vi "PantherLAB_Log - Rename DQMH Event.vi"(9 "New Event Name":string, 10 "Event Info (Existing)":T1={"Event VI Path"=path "", "Argument Path"=path "", "Wait Argument Path"=path "", "Event Arg Owner"=-1, "Event Name"="", "Type"=enum."Request"}, 11 "Module Info":T3) -> (0 "error out":errorcluster)   [LabVIEW 2016]
doc: "_____\nCreated using DQMH Framework: Event Scripter 7.1.0.1450."
uses:
  <vilib>/Delacor/Delacor QMH/Libraries/_Scripting Support/Module Info--cluster.ctl
  <vilib>/Delacor/Delacor QMH/Libraries/_Scripting Support/Module Type--enum.ctl
  <vilib>/Delacor/Delacor QMH/Libraries/_Scripting Support/Event Info (Existing)--cluster.ctl
  Program Files (x86)/National Instruments/LabVIEW 2016/project/Delacor/DQMH/_DQMH Remove Event/Event Type (All Permutations)--enum.ctl
  PantherLAB Scripting Hooks/PantherLAB_Log.lvlib
  <vilib>/Delacor/Delacor QMH/Libraries/_Scripting Support/dqmh_lib_DQMH Scripting Support.lvlib
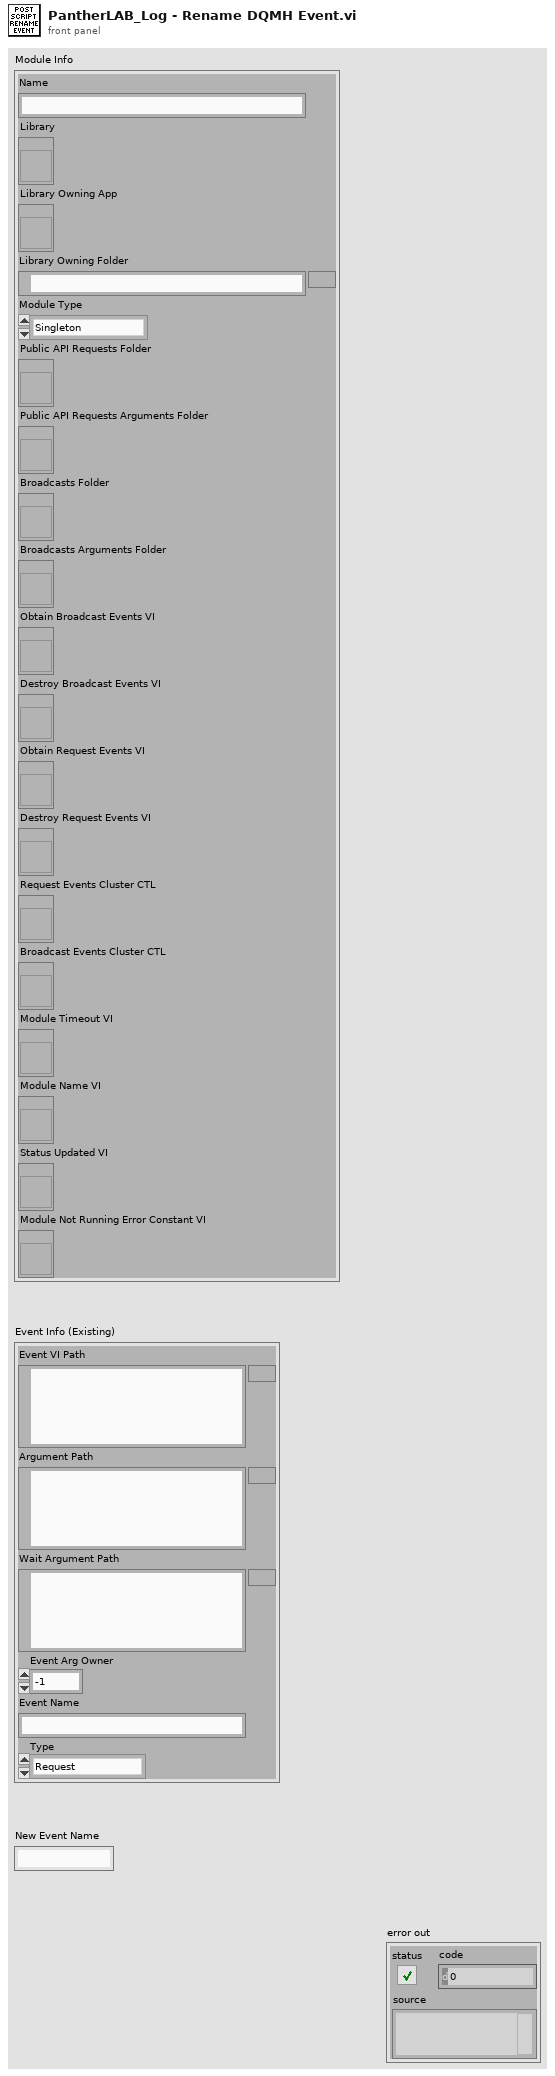
[diagram p1: front panel]
types:
  T1 = typedef "dqmh_lib_DQMH Scripting Support.lvlib/Event Info (Existing)--cluster.ctl" = cluster{"Event VI Path":path, "Argument Path":path, "Wait Argument Path":path, "Event Arg Owner":i32, "Event Name":string, "Type":T2}
  T2 = typedef "dqmh_lib_DQMH Scripting Support.lvlib/Event Type (All Permutations)--enum.ctl" = enum16{"Request", "Broadcast", "Both", "Request (no Wait)", "Request and Wait", "Request (Private)", "Request (Local Instance)"}
  T3 = typedef "dqmh_lib_DQMH Scripting Support.lvlib/Module Info--cluster.ctl" = cluster{"Name":string, "Library":refnum<vi>, "Library Owning App":refnum<vi>, "Library Owning Folder":path, "Module Type":T4, "Public API Requests Folder":refnum<vi>, "Public API Requests Arguments Folder":refnum<vi>, "Broadcasts Folder":refnum<vi>, "Broadcasts Arguments Folder":refnum<vi>, "Obtain Broadcast Events VI":refnum<vi>, "Destroy Broadcast Events VI":refnum<vi>, "Obtain Request Events VI":refnum<vi>, "Destroy Request Events VI":refnum<vi>, "Request Events Cluster CTL":refnum<vi>, "Broadcast Events Cluster CTL":refnum<vi>, "Module Timeout VI":refnum<vi>, "Module Name VI":refnum<vi>, "Status Updated VI":refnum<vi>, "Module Not Running Error Constant VI":refnum<vi>}
  T4 = typedef "dqmh_lib_DQMH Scripting Support.lvlib/Module Type--enum.ctl" = enum16{"Singleton", "Cloneable"}
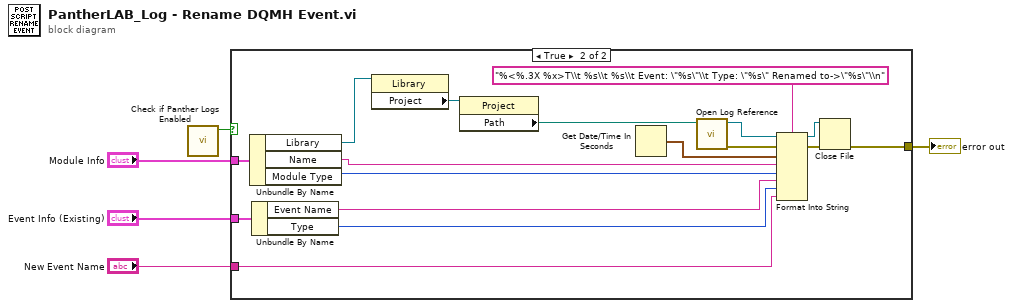
[diagram p0: block diagram]
diagram:
  n1 = call "Check if Panther Logs Enabled.vi"() -> ("PantherLogs Enabled?"=w4:bool)  [unwired: 11 in]
  n2 = case shown="True" w4 {
    tunnel: [_ w20] -> w5
    tunnel: "Module Info" -> [_ w19]
    tunnel: "New Event Name" -> [_ w7]
    tunnel: "Event Info (Existing)" -> [_ w10]
    frame False {
    }
    frame True {
      n3 = Unbundle By Name(w19) -> ("Library"=w18:refnum<vi>, "Name"=w14:string, "Module Type"=w13:T4)
      n4 = Unbundle By Name(w10) -> ("Event Name"=w9:string, "Type"=w8:T2)
      n5 = property class="Library"(reference=w18) -> ("Project"=w17:refnum<vi>)  [unwired: 1 in, 2 out]
      n6 = property class="Project"(reference=w17) -> ("Path"=w11:path)  [unwired: 1 in, 2 out]
      n7 = Get Date/Time In Seconds() -> (seconds since 1Jan1904=w12:timestamp)
      n8 = call "Open Log Reference.vi"("Project Path"=w11) -> ("error out"=w22:errorcluster, "File Reference"=w16:refnum<file>)  [unwired: 9 in]
      n9 = Format Into String(format string="%<%.3X %x>T\\t %s\\t %s\\t Event: \"%s\"\\t Type: \"%s\" Renamed to->\"%s\"\\n", initial string=w16, error in=w22, w12, w14, w13, w9, w8, w7) -> (resulting string=w15:refnum<file>, error out=w21:errorcluster)
      n10 = Close File(refnum=w15, error in=w21) -> (error out=w20:errorcluster)  [unwired: 1 out]
    }
  }
  "error out" <- w5
